vi "write_data.vi"(8 "error in (no error)":errorcluster, 10 "data":T1, 11 "SVM in":refnum<class "SVM.lvclass">) -> (0 "error out":errorcluster, 3 "SVM out":refnum<class "SVM.lvclass">)   [LabVIEW 2020, in "SVM.lvclass"]
uses:
  SVM.lvclass
  Controls/svm_data.ctl
  SVM.lvclass/SVM.ctl
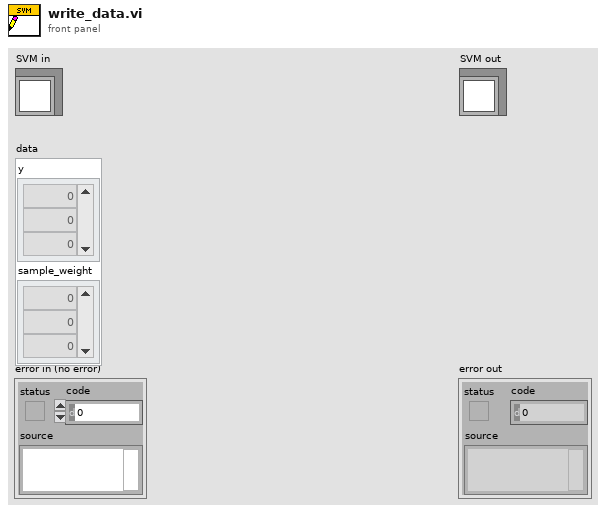
[diagram p1: front panel]
types:
  T1 = typedef "svm_data.ctl" = cluster{"y":dbl[], "sample_weight":dbl[]}
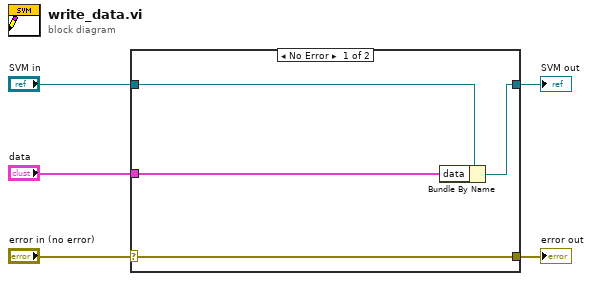
[diagram p0: block diagram]
diagram:
  n1 = case shown="No Error" "error in (no error)" {
    selector: "error in (no error)" -> [w9 w10]
    tunnel: [w9 w10] -> w4
    tunnel: [w7 w11] -> w2
    tunnel: "SVM in" -> [w8 w11]
    tunnel: "data" -> [w6 _]
    frame No Error {
      n2 = Bundle By Name(cluster=w8, "data"=w6) -> (w7:refnum<class "SVM.lvclass">)
    }
    frame Error {
    }
  }
  "error out" <- w4
  "SVM out" <- w2
